vi "Delete.vi"(8 "error in (no error)":errorcluster, 11 "LabVIEW-Config.lvlib:LabVIEW-Config.lvclass":refnum<class "LabVIEW-Config.lvclass">) -> (0 "error out":errorcluster, 1 "Modified?":bool, 2 "Text":string, 3 "Path":path)   [LabVIEW 2017, in "LabVIEW-Config.lvlib" / "LabVIEW-Config.lvclass"]
uses:
  LabVIEW-Config.lvclass
  LabVIEW-Config.lvclass/LabVIEW-Config.ctl
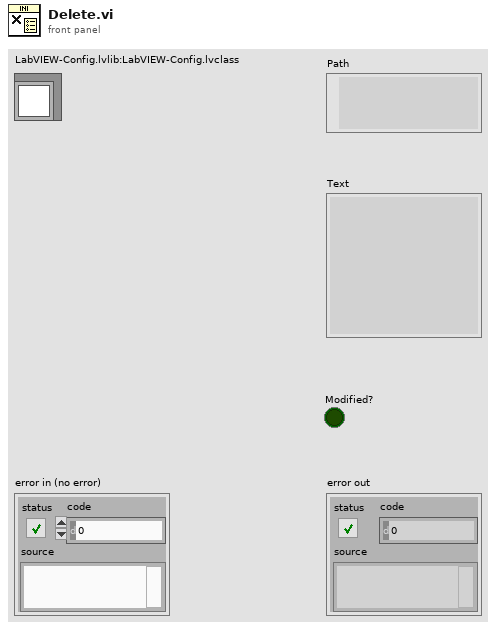
[diagram p1: front panel]
types:
  T1 = typedef "LabVIEW-Config.lvlib/LabVIEW-Config.lvclass/LineToken.ctl" = enum8{"comment", "section", "key", "more"}
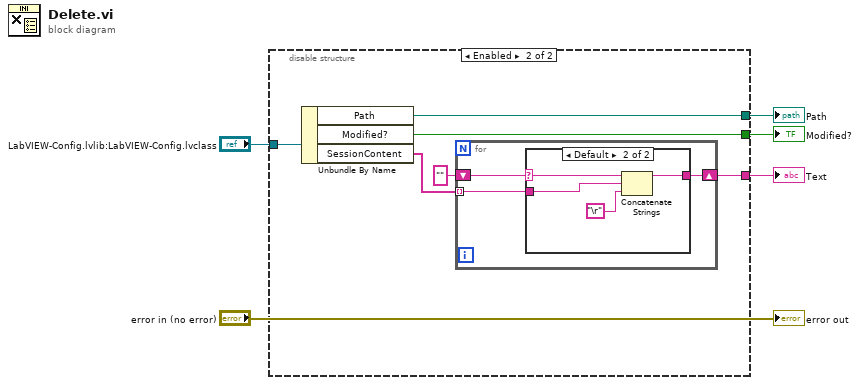
[diagram p0: block diagram]
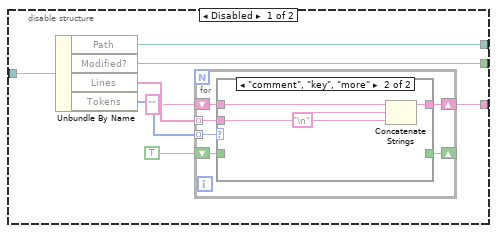
[diagram p2: hidden frame]
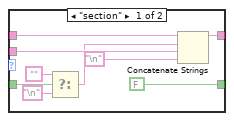
[diagram p3: hidden frame]
diagram:
  n1 = disable-structure shown="Enabled" {
    disable-tunnel: "LabVIEW-Config.lvlib:LabVIEW-Config.lvclass" -> [w13 w38]
    disable-tunnel: [w10 w36] -> w3
    disable-tunnel: [w7 w34] -> w2
    disable-tunnel: [w6 w33] -> w1
    frame Disabled {
      n2 = Unbundle By Name(w13) -> ("Path"=w10:path, "Modified?"=w7:bool, "Lines"=w12:string[], "Tokens"=w11:T1[])
      n3 = for {
        tunnel: w12 -> [w17] mode=indexing
        tunnel: w11 -> [w19] mode=indexing
        shift-right: [w18] -> w6
        shift-left: "" -> [w16]
        shift-right: [w14] -> _
        shift-left: TRUE -> [w15]
        n4 = case shown="\"comment\", \"key\", \"more\"" w19 {
          tunnel: [w27 w31] -> w18
          tunnel: w17 -> [w28 w32]
          tunnel: w16 -> [w25 w29]
          tunnel: w15 -> [w23 _]
          tunnel: [FALSE _] -> w14
          frame "section" {
            n5 = Select(t="" ("Empty String Constant"), s=w23, f="\n" ("Line Feed Constant")) -> (s? t:f=w21:string)
            n6 = Concatenate Strings(w25, w21, w28, "\n" ("Line Feed Constant")) -> (w27:string)
          }
          frame "comment", "key", "more" {
            n7 = Concatenate Strings(w29, w32, "\n" ("Line Feed Constant")) -> (w31:string)
          }
        }
      }
    }
    frame Enabled {
      n8 = Unbundle By Name(w38) -> ("Path"=w36:path, "Modified?"=w34:bool, "SessionContent"=w37:string[])
      n9 = for {
        tunnel: w37 -> [w40] mode=indexing
        shift-right: [w41] -> w33
        shift-left: "" -> [w39]
        n10 = case shown="Default" w39 {
          selector: w39 -> [_ w44]
          tunnel: [w42 w46] -> w41
          tunnel: w40 -> [w42 w45]
          frame "" {
          }
          frame Default {
            n11 = Concatenate Strings(w44, w45, "\r") -> (w46:string)
          }
        }
      }
    }
  }
  "Path" <- w3
  "Modified?" <- w2
  "Text" <- w1
  "error out" <- "error in (no error)"
